vi "Initialize.vi"(8 "error in":errorcluster, 10 "parameters":variant, 11 "ACIR Instrument":refnum<class "ACIR Instrument.lvclass">) -> (0 "error out":errorcluster, 2 "summary":T2[](array[typedef]), 3 "data value reference":T1)   [LabVIEW 2025, in "ACIR.lvlib" / "ACIR Instrument.lvclass"]
doc: "Initializes the data of a node to its default state.\nThe object is not created inside of this VI, because it is created from a File depending on user selection.\nCopyright 2017 National Instruments Corporation\n\nLicensed under the Apache License, Version 2.0 (the \"License\"); you may not use this file except in compliance with the License. You may obtain a copy of the License at http://www.apache.org/licenses/LICENSE-2.0\nUnless required by applicable law or agreed to in writing, software distributed under the License is distributed on an \"AS IS\" BASIS, WITHOUT WARRANTIES OR CONDITIONS OF ANY KIND, either express or implied. See the License for the specific language governing permissions and limitations under the License."
uses:
  ACIR Instrument.lvclass
  Users/Public/Documents/Sandia National Labs/TSS Plugin/CEF.lvlibp/Node/Summary.ctl
  Users/Public/Documents/Sandia National Labs/TSS Plugin/CEF.lvlibp/Node/NodeRef.ctl
  Users/Public/Documents/Sandia National Labs/TSS Plugin/CEF.lvlibp/Node/CEF_Node.lvclass
  ACIR Instrument.lvclass/ACIR Instrument.ctl
  ACIR configuration/ACIR configuration.lvclass
  C:/Users/Public/Documents/Sandia National Labs/TSS Plugin/Abstract Engine.lvlibp/Instrument configuration/Instrument configuration.lvclass
  Users/Public/Documents/Sandia National Labs/TSS Plugin/Abstract Engine.lvlibp/Instrument configuration/Read Instrument Setting.vi
  Users/Public/Documents/Sandia National Labs/TSS Plugin/Abstract Engine.lvlibp/Instrument configuration/Write Instrument Setting.vi
  Users/Public/Documents/Sandia National Labs/TSS Plugin/Abstract Engine.lvlibp/Abstract Instrument/Abstract Instrument.lvclass
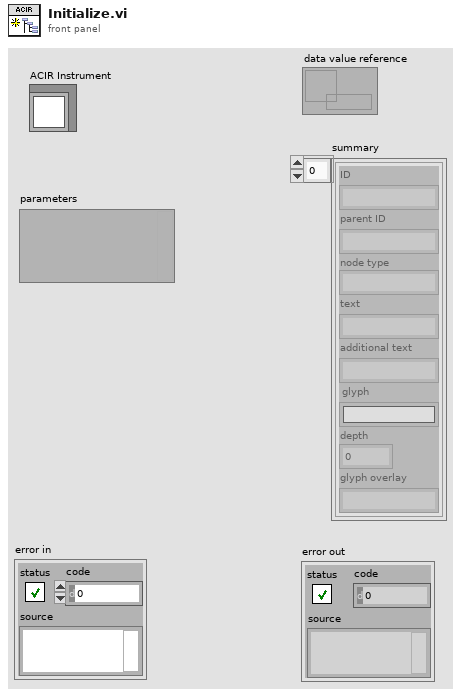
[diagram p1: front panel]
types:
  T1 = typedef "CEF.lvlibp/CEF_Node.lvclass/NodeRef.ctl" = refnum<data-value>
  T2 = typedef "CEF.lvlibp/CEF_Node.lvclass/Summary.ctl" = cluster{"ID":string, "parent ID":string, "node type":string, "text":string, "additional text":string, "glyph":string, "depth":i32, "glyph overlay":string}
  T3 = typedef "Abstract Engine.lvlibp/Instrument configuration.lvclass/Default Instrument.ctl" = cluster{"Type":string, "Address":string, "SW Alias":string, "Description":string, "Enabled":bool}
  T4 = cluster{"ID":string, "parent ID":string, "node type":string, "text":string, "additional text":string, "glyph":string, "depth":i32, "glyph overlay":string}[]
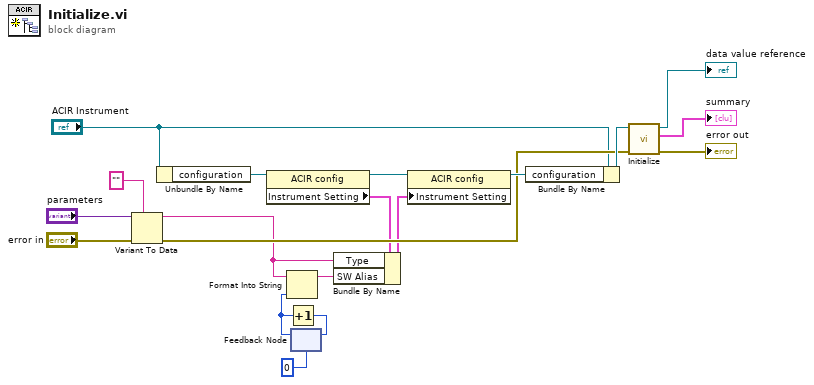
[diagram p0: block diagram]
diagram:
  n1 = Variant To Data(error in="error in", type="", Variant="parameters") -> (data=w1:string, error out=w10:errorcluster)
  n2 = Unbundle By Name("ACIR Instrument") -> ("configuration"=w12:refnum<class "ACIR configuration.lvclass">)
  n3 = property class="ACIR config"(reference=w12) -> (reference out=w11:refnum<class "ACIR configuration.lvclass">, "Instrument Setting"=w8:T3)  [unwired: 1 in, 1 out]
  n4 = feedback #1(0) -> (w6:i32)
  n5 = Format Into String(initial string=w1, w6) -> (resulting string=w3:string)  [unwired: 2 in, 1 out]
  n6 = Increment(x=w6) -> (x+1=w4:i32)
  n7 = feedback-in #1(w4) -> ()
  n8 = Bundle By Name(cluster=w8, "Type"=w1, "SW Alias"=w3) -> (w7:T3)
  n9 = property class="ACIR config"(reference=w11, "Instrument Setting"=w7) -> (reference out=w14:refnum<class "ACIR configuration.lvclass">)  [unwired: 1 in, 1 out]
  n10 = Bundle By Name(cluster="ACIR Instrument", "configuration"=w14) -> (w15:refnum<class "ACIR Instrument.lvclass">)
  n11 = call-parent "Initialize.vi"("error in"=w10, "CEF_Serialize node in"=w15) -> ("error out"=→"error out":errorcluster, "summary"=→"summary":T4, "data value reference"=→"data value reference":refnum<data-value>)  [unwired: 7 in]
